vi "Main_010.vi"() -> ()   [LabVIEW 2025]
uses:
  Utility/Universal Utility/TypeDefs_Utility/Cluster_Row-Column.ctl
  9e3f57c0-2ef8-4495-8287-c6a42a5fb955.vi
  Utility/Universal Utility/TypeDefs_Utility/ENUM_4 Directions U-D-L-R.ctl
  Utility/Universal Utility/TypeDefs_Utility/ENUM_8 Directions U-D-L-R.ctl
  <vilib>/gmath/NI_AAL_MathFunc.lvlib
panel:
  out "MATCH":bool
  in  "Select Data":enum32{"Example", "Puzzle"}(tab)
  in  "EX Target":u64=17
  in  "Example Input":u64=10
  in  "Puzzle Input":u64=2000000
  in  "Puzzle Target":u64=142913828922
  out "Answer":u64
  # "Sum of Primes Below X"
  # "Sum of Primes"
  # "Sum of Primes"
  # "Sum of Primes Below X"
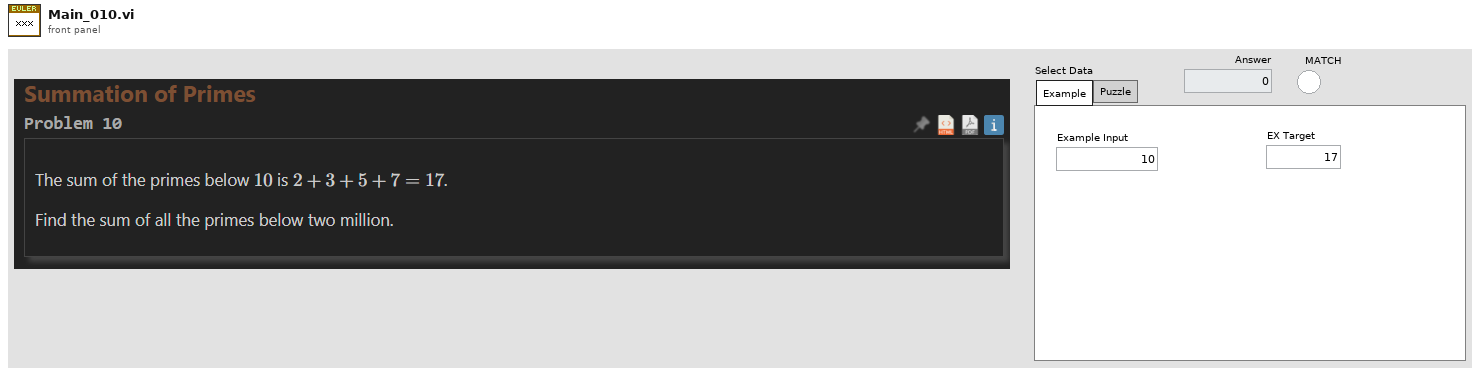
[diagram p1: front panel]
types:
  T1 = typedef "ENUM_8 Directions U-D-L-R.ctl" = enum16{"Up;-1,0", "Up-Right;-1,1", "Right;0,1", "Down-Right;1,1", "Down;1,0", "Down-Left;1,-1", "Left;0,-1", "Up-Left;-1,-1"}
  T2 = typedef "ENUM_4 Directions U-D-L-R.ctl" = enum16{"Up;-1,0", "Right;0,1", "Down;1,0", "Left;0,-1"}
  T3 = typedef "Cluster_Row-Column.ctl" = cluster{"R":i32, "C":i32}
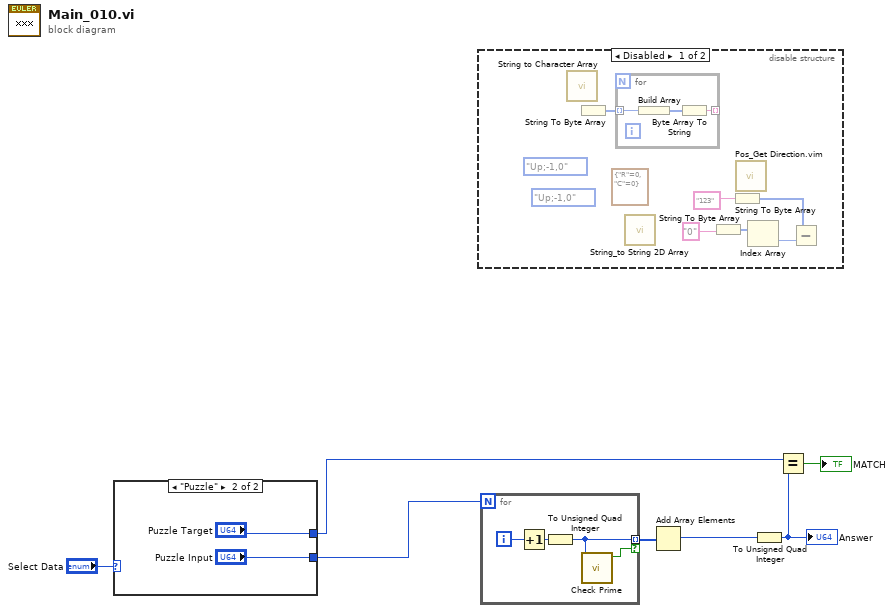
[diagram p0: block diagram]
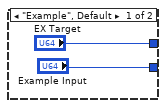
[diagram p2: hidden frame]
diagram:
  n1 = case shown="\"Puzzle\"" "Select Data" {
    tunnel: ["Example Input" "Puzzle Input"] -> w3
    tunnel: ["EX Target" "Puzzle Target"] -> w5
    frame "Example", Default {
    }
    frame "Puzzle" {
    }
  }
  n2 = disable-structure shown="Disabled" {
    frame Disabled {
      (unwired) ENUM_8_Directions_U-D-L-R."Up;-1,0" ("Direction 8")
      (unwired) ENUM_4_Directions_U-D-L-R."Up;-1,0" ("Direction")
      (unwired) T3 {"R"=0, "C"=0} ("Position")
      n3 = call "String to Character Array.vi"() -> ()  [unwired: 1 in, 1 out]
      n4 = String To Byte Array() -> (unsigned byte array=w12:u8[])  [unwired: 1 in]
      n5 = for {
        tunnel: w12 -> [w20] mode=indexing
        tunnel: [w18] -> _ mode=indexing
        n6 = Build Array(w20) -> (w19:u8[])
        n7 = Byte Array To String(unsigned byte array=w19) -> (string=w18:string)
      }
      n8 = call "String_to String 2D Array.vi"() -> ()  [unwired: 11 in, 1 out]
      n9 = String To Byte Array(string="0") -> (unsigned byte array=w15:u8[])
      n10 = String To Byte Array(string="123") -> (unsigned byte array=w13:u8[])
      n11 = call "Pos_Get Direction.vim"() -> ()  [unwired: 11 in, 1 out]
      n12 = Index Array(array=w15) -> (element=w14:u8)  [unwired: 1 in]
      n13 = Subtract(x=w13, y=w14) -> ()  [unwired: 1 out]
    }
    frame Enabled {
    }
  }
  n14 = for {
    N: w3 -> [_]
    tunnel: [w22] -> w2 mode=indexing if=w21
    i -> [w24]
    n15 = Increment(x=w24) -> (x+1=w23:i32)
    n16 = To Unsigned Quad Integer(1:w23) -> (0:w22:u64)
    n17 = call <vilib>:"Check Prime.vi"("n"=w22) -> ("prime?"=w21:bool)  [unwired: 10 in]
  }
  n18 = Add Array Elements(numeric array=w2) -> (sum=w1:u64)
  n19 = To Unsigned Quad Integer(1:w1) -> (0:w4:u64)
  "Answer" <- w4
  n20 = Equal?(x=w5, y=w4) -> (x = y?=→"MATCH":bool)
